vi "RGB to CMYK.vi"(0 "Red":u8, 5 "Green":u8, 7 "Blue":u8, 11 "error in (no error)":errorcluster) -> (4 "Cyan(%)":dbl format="%#.2g", 6 "Magenta(%)":dbl format="%#.2g", 8 "Yellow(%)":dbl format="%#.2g", 10 "Key/Black(%)":dbl format="%#.2g", 15 "error out":errorcluster)   [LabVIEW 2018, in "Colour Lab.lvlib"]
uses:
  Colour Lab.lvlib
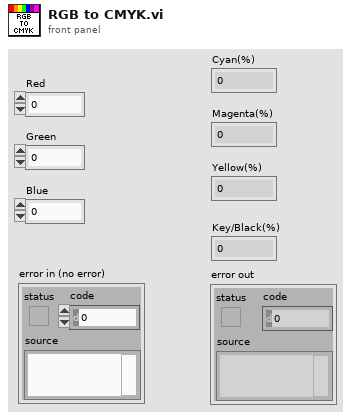
[diagram p1: front panel]
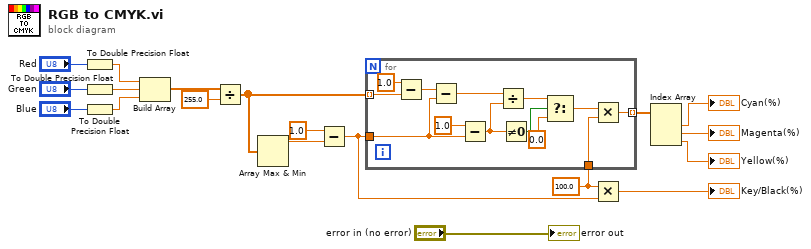
[diagram p0: block diagram]
diagram:
  w3 = 100.0 ("y")
  n1 = To Double Precision Float(number="Red") -> (double precision float=w13:dbl)
  n2 = To Double Precision Float(number="Green") -> (double precision float=w14:dbl)
  n3 = To Double Precision Float(number="Blue") -> (double precision float=w15:dbl)
  n4 = Build Array(w13, w14, w15) -> (w12:dbl[])
  n5 = Divide(x=w12, y=255.0) -> (x/y=w8:dbl[])
  n6 = Array Max & Min(array=w8) -> (max value=w10:dbl)  [unwired: 3 out]
  n7 = Subtract(x=1.0, y=w10) -> (x-y=w5:dbl)
  n8 = for {
    tunnel: w8 -> [w22] mode=indexing
    tunnel: w5 -> [w31]
    tunnel: [w29] -> w7 mode=indexing
    tunnel: w3 -> [w28]
    n9 = Subtract(x=1.0, y=w22) -> (x-y=w32:dbl)
    n10 = Subtract(x=w32, y=w31) -> (x-y=w20:dbl)
    n11 = Subtract(x=1.0, y=w31) -> (x-y=w27:dbl)
    n12 = Divide(x=w20, y=w27) -> (x/y=w25:dbl)
    n13 = Not Equal To 0?(x=w27) -> (x != 0?=w26:bool)
    n14 = Select(t=w25, s=w26, f=0.0) -> (s? t:f=w23:dbl)
    n15 = Multiply(x=w23, y=w28) -> (x*y=w29:dbl)
  }
  n16 = Multiply(x=w3, y=w5) -> (x*y=→"Key/Black(%)":dbl)
  n17 = Index Array(array=w7) -> (element #1=→"Cyan(%)":dbl, element #2=→"Magenta(%)":dbl, element #3=→"Yellow(%)":dbl)  [unwired: 3 in]
  "error out" <- "error in (no error)"
